vi "numeric_array_to_sreadsheet_file.vi"() -> ()   [LabVIEW 2015]
panel:
  out "Array":i32[][](array[numeric])
  out "spreadsheet string":string
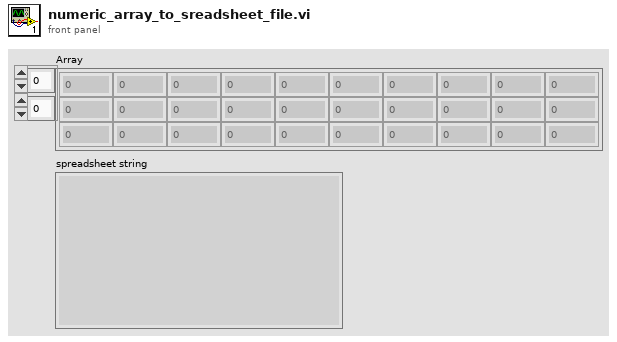
[diagram p1: front panel]
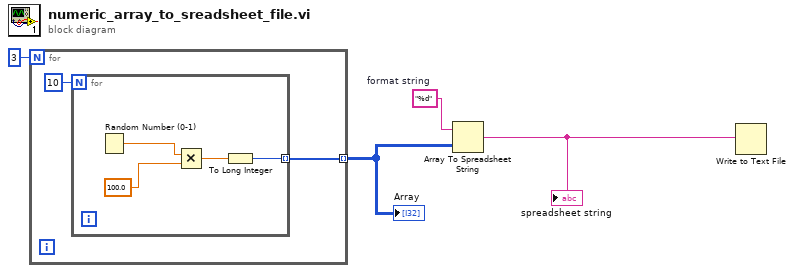
[diagram p0: block diagram]
diagram:
  w4 = "%d"  # format string
  n1 = for {
    N: 3 -> [_]
    tunnel: [w5] -> w1 mode=indexing
    n2 = for {
      N: 10 -> [_]
      tunnel: [w7] -> w5 mode=indexing
      n3 = Random Number (0-1)() -> (number: 0 to 1=w8:dbl)
      n4 = Multiply(x=w8, y=100.0) -> (x*y=w9:dbl)
      n5 = To Long Integer(number=w9) -> (32bit integer=w7:i32)
    }
  }
  "Array" <- w1
  n6 = Array To Spreadsheet String(array=w1, 3:w4) -> (spreadsheet string=w3:string)  [unwired: 1 in]
  "spreadsheet string" <- w3
  n7 = Write to Text File(text=w3) -> ()  [unwired: 3 in, 3 out]
